vi "Waveform.vi"() -> ()   [LabVIEW 2011]
uses:
  <vilib>/FPGAPlugInAG/sbRIO-9606/niLvFpga_Open_sbRIO-9606.vi
  <vilib>/FPGAPlugInAG/sbRIO-9606/niLvFpga_Run_sbRIO-9606.vi
  <vilib>/Utility/error.llb/Error Cluster From Error Code.vi
  <vilib>/rvi/errors/niLvFpgaAdjustHostInterfaceError.vi
  <vilib>/rvi/interface/nirviOpenFPGA/nirviOpenFPGA.xnode
  FPGA Bitfiles/JAGM_FPGATarget_TestChan1_9C6359DC.lvbitx
  <vilib>/rvi/interface/nirviMethod/nirviMethod.xnode
  <vilib>/rvi/interface/nirviReadWriteControl/nirviReadWriteControl.xnode
  NiFpgaLv.dll
panel:
  in  "Enable_RE":bool
  in  "Enable_ON":bool=TRUE
  out "Waveform Chart 2":i16(graph)
  out "Waveform Chart":i16(graph)
  in  "stop":bool
  out "error out":errorcluster
  in  "error in (no error)":errorcluster
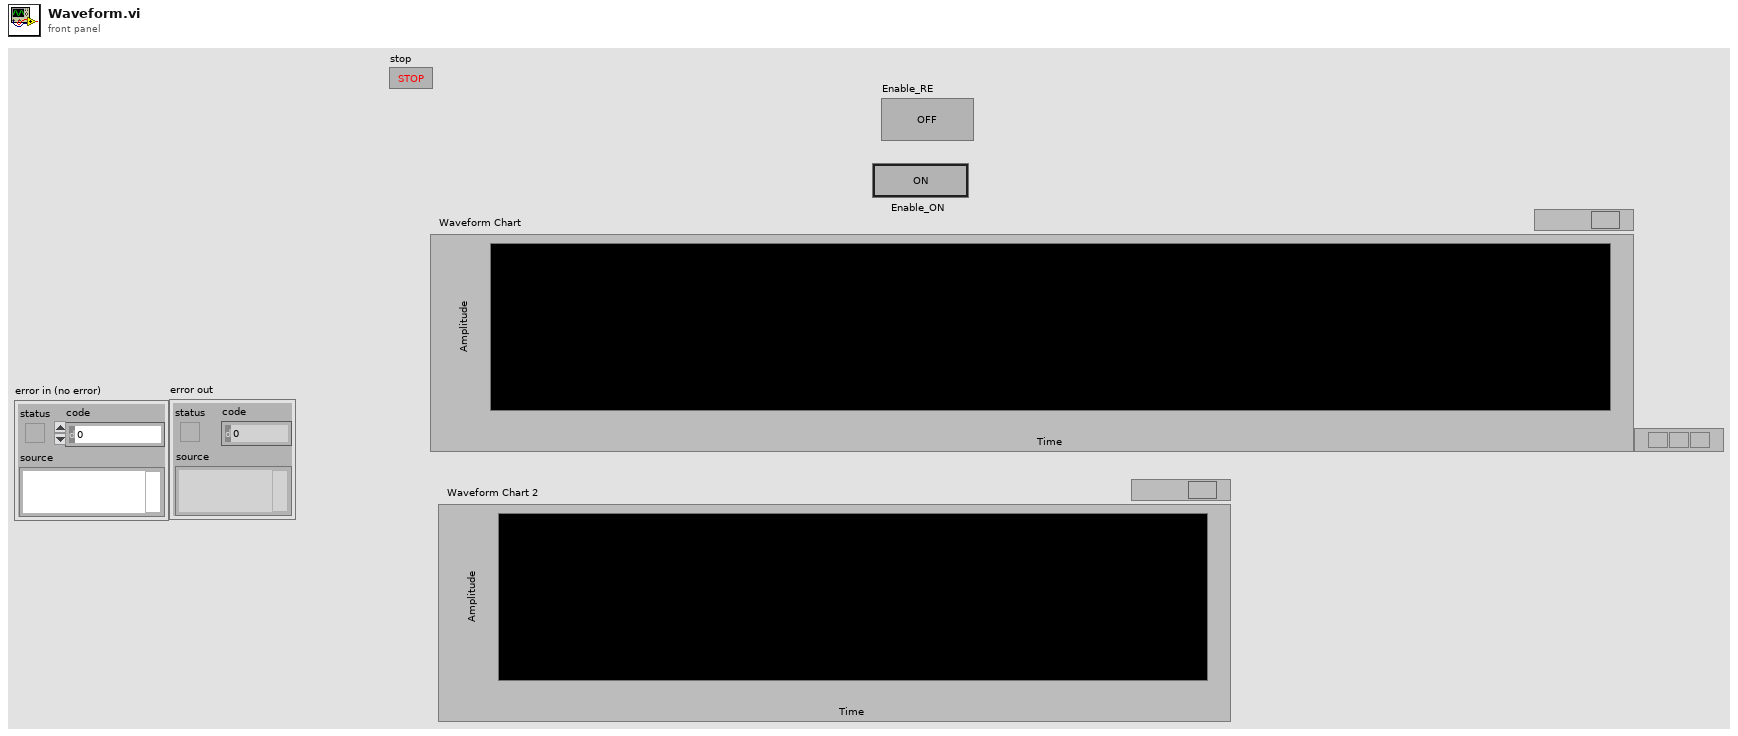
[diagram p1: front panel]
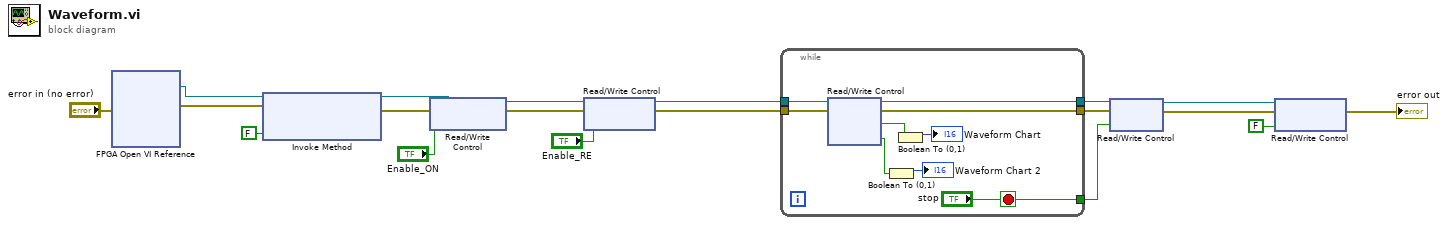
[diagram p0: block diagram]
diagram:
  n1 = xnode "FPGA Open VI Reference"("error in"="error in (no error)") -> ("FPGA VI Reference Out"=w8:refnum<k20>, "error out"=w7:errorcluster)  [unwired: 1 in]
  n2 = xnode "Invoke Method"("FPGA VI Reference In"=w8, "error in"=w7, "Wait Until Done (F)"=FALSE) -> ("FPGA VI Reference Out"=w10:refnum<k20>, "error out"=w9:errorcluster)
  n3 = xnode "Read/Write Control"("FPGA VI Reference In"=w10, "error in"=w9, "Enable_ON"="Enable_ON") -> ("FPGA VI Reference Out"=w5:refnum<k20>, "error out"=w3:errorcluster)
  n4 = xnode "Read/Write Control"("FPGA VI Reference In"=w5, "error in"=w3, "Enable_RE"="Enable_RE") -> ("FPGA VI Reference Out"=w4:refnum<k20>, "error out"=w2:errorcluster)
  n5 = while {
    tunnel: w4 -> [w28]
    tunnel: w2 -> [w27]
    tunnel: [w26] -> w16
    tunnel: [w25] -> w17
    tunnel: ["stop"] -> w15
    stop <- "stop" stop-if-true
    n6 = xnode "Read/Write Control"("FPGA VI Reference In"=w28, "error in"=w27) -> ("FPGA VI Reference Out"=w25:refnum<k20>, "error out"=w26:errorcluster, "Signal"=w21:bool, "Clk"=w20:bool)
    n7 = Boolean To (0,1)(Boolean=w20) -> (0, 1=→"Waveform Chart 2":i16)
    n8 = Boolean To (0,1)(Boolean=w21) -> (0, 1=→"Waveform Chart":i16)
  }
  n9 = xnode "Read/Write Control"("FPGA VI Reference In"=w17, "error in"=w16, "Stop"=w15) -> ("FPGA VI Reference Out"=w14:refnum<k20>, "error out"=w13:errorcluster)
  n10 = xnode "Read/Write Control"("FPGA VI Reference In"=w14, "error in"=w13, "Enable_RE"=FALSE ("Enable")) -> ("error out"=→"error out":errorcluster)  [unwired: 1 out]
